vi "UTS - Character Count Limit Exceeded.vi"(9 "Include Buffer":bool, 10 "Character Count Limit":i32, 11 "Response String in":string) -> (2 "Limit Exceeded":bool)   [LabVIEW 2017, in "SSH.lvlib"]
doc: "Sets the buffer length to 5 to enable testing"
uses:
  SSH.lvlib
  Character Count Configuration.ctl
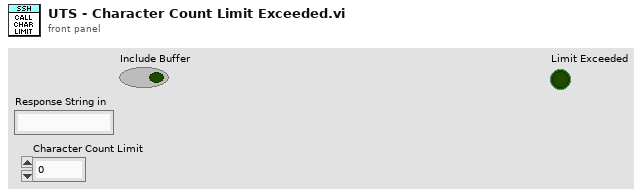
[diagram p1: front panel]
types:
  T1 = typedef "SSH.lvlib/Character Count Configuration.ctl" = cluster{"Character Count Limit":i32, "Include Buffer":bool}
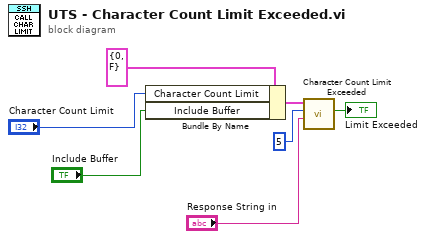
[diagram p0: block diagram]
diagram:
  n1 = Bundle By Name(cluster=T1 {"Character Count Limit"=0, "Include Buffer"=FALSE} ("Character Count Configuration"), "Character Count Limit"="Character Count Limit", "Include Buffer"="Include Buffer") -> (w3:T1)
  n2 = call "Character Count Limit Exceeded.vi"("Response String in"="Response String in", "Buffer Length"=5, "Character Count Configuration"=w3) -> ("Limit Exceeded"=→"Limit Exceeded":bool)  [unwired: 8 in]
